vi "plot_dataSubset.vi"(1 "spectrum property":T2, 3 "zoom range low":ext format="%.2f", 4 "zoom range high":sgl format="%.2f", 5 "error in (no error)":errorcluster) -> (14 "idx start":i32, 15 "length":i32, 17 "X min actual":sgl format="%.2f", 18 "X max actual":sgl format="%.2f", 19 "error out":errorcluster)   [LabVIEW 2010, in "OSA.lvclass"]
doc: "SubVI to a <B>Thorlabs_OSA_64</B> object.\n\n[GOOP 1.0]"
uses:
  OSA.lvclass
  typeDef/xVal_option.ctl
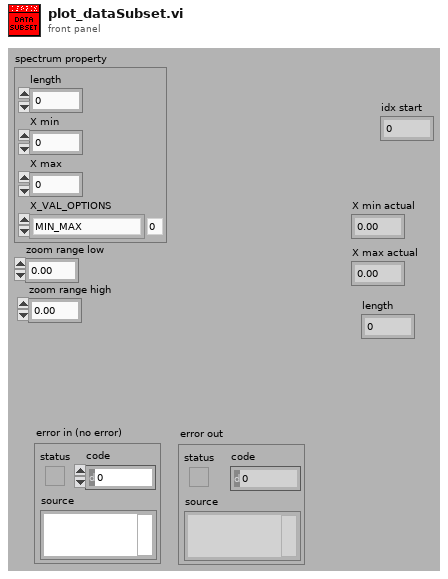
[diagram p1: front panel]
types:
  T1 = typedef "OSA.lvclass/xVal_option.ctl" = enum16{"MIN_MAX", "ARRAY"}
  T2 = cluster{"length":u32, "X min":sgl, "X max":sgl, "X_VAL_OPTIONS":T1}
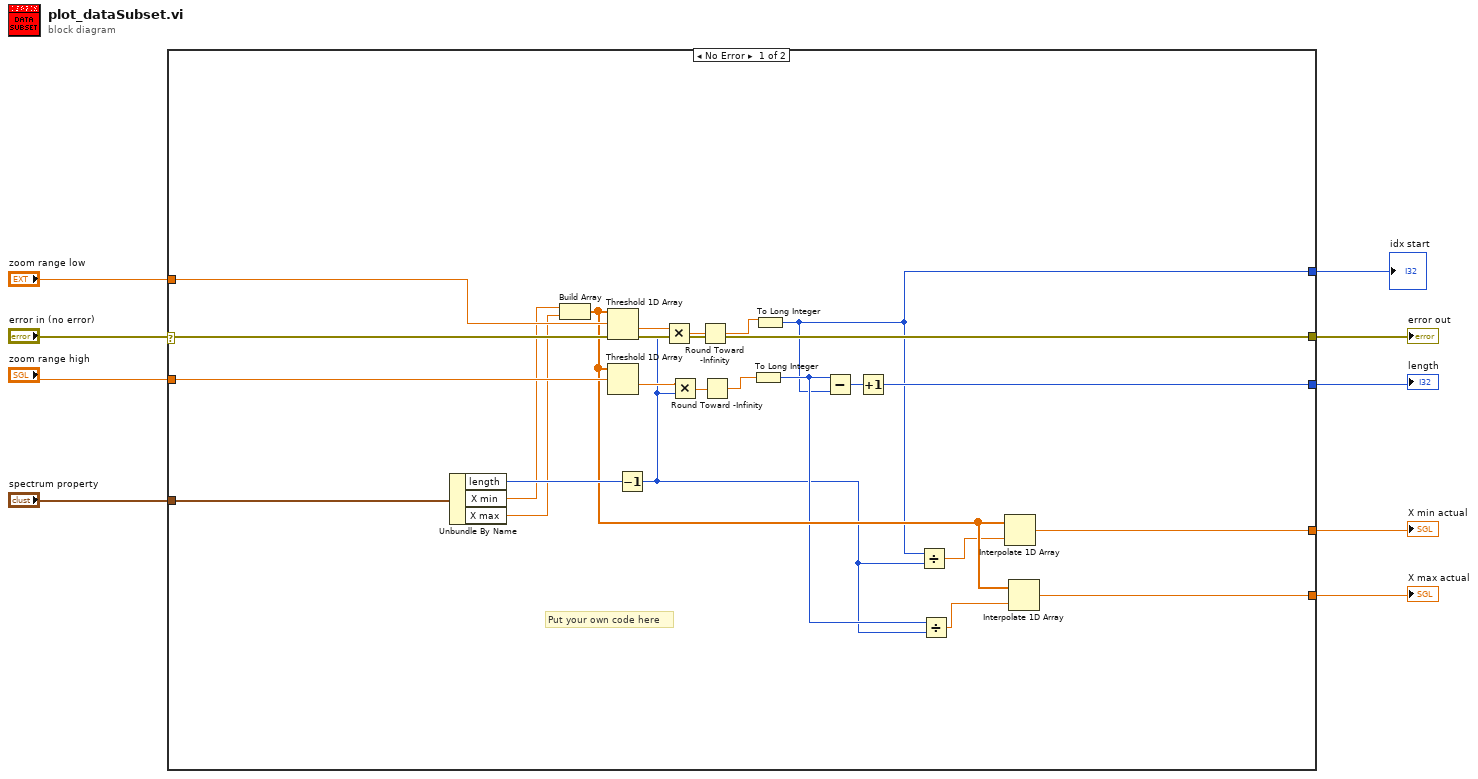
[diagram p0: block diagram]
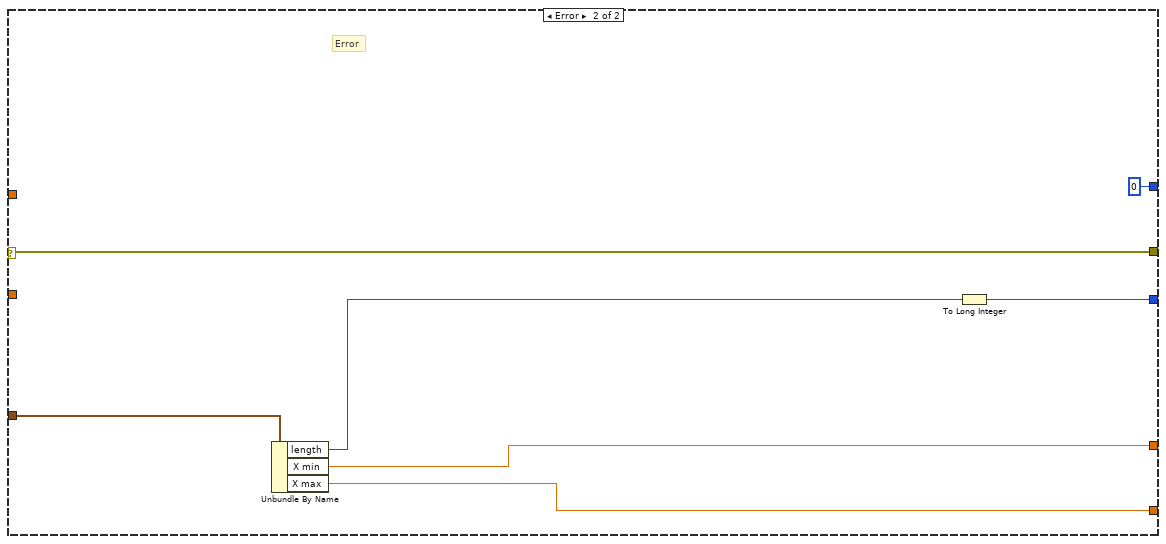
[diagram p2: hidden frame]
diagram:
  n1 = case shown="No Error" "error in (no error)" {
    selector: "error in (no error)" -> [w32 w39]
    tunnel: [w32 w39] -> w9
    tunnel: "spectrum property" -> [w26 w38]
    tunnel: "zoom range low" -> [w25 _]
    tunnel: "zoom range high" -> [w24 _]
    tunnel: [w14 w35] -> w4
    tunnel: [w11 w33] -> w3
    tunnel: [w15 w36] -> w2
    tunnel: [w10 0] -> w1
    frame No Error {
      # "Put your own code here"
      n2 = Unbundle By Name(w26) -> ("length"=w29:u32, "X min"=w19:sgl, "X max"=w20:sgl)
      n3 = Build Array(w19, w20) -> (w21:sgl[])
      n4 = Threshold 1D Array(2:w25, 3:w21) -> (0:w31:sgl)  [unwired: 1 in]
      n5 = Threshold 1D Array(2:w24, 3:w21) -> (0:w30:sgl)  [unwired: 1 in]
      n6 = Decrement(x=w29) -> (x-1=w12:u32)
      n7 = Multiply(x=w31, y=w12) -> (x*y=w28:sgl)
      n8 = Multiply(x=w30, y=w12) -> (x*y=w27:sgl)
      n9 = Round Toward -Infinity(1:w28) -> (0:w23:sgl)
      n10 = Round Toward -Infinity(1:w27) -> (0:w22:sgl)
      n11 = To Long Integer(number=w22) -> (32bit integer=w16:i32)
      n12 = To Long Integer(number=w23) -> (32bit integer=w10:i32)
      n13 = Subtract(x=w16, y=w10) -> (x-y=w13:i32)
      n14 = Increment(x=w13) -> (x+1=w11:i32)
      n15 = Divide(x=w10, y=w12) -> (x/y=w18:dbl)
      n16 = Divide(x=w16, y=w12) -> (x/y=w17:dbl)
      n17 = Interpolate 1D Array(1:w18, 2:w21) -> (0:w15:sgl)
      n18 = Interpolate 1D Array(1:w17, 2:w21) -> (0:w14:sgl)
    }
    frame Error {
      # "Error"
      n19 = Unbundle By Name(w38) -> ("length"=w37:u32, "X min"=w36:sgl, "X max"=w35:sgl)
      n20 = To Long Integer(number=w37) -> (32bit integer=w33:i32)
    }
  }
  "error out" <- w9
  "X min actual" <- w2
  "X max actual" <- w4
  "length" <- w3
  "idx start" <- w1
